vi "Explore_Volume.vi"(5 "Traverse line In":T1 {"Carrier_2 Q (l/min)" format="%#.2f"; "Row Duration (mins)" format="%#.1f"; "Row No" min=0; "Trace Gas Concentration (%)" min=0.0 format="%#_4f"; "Carrier_1 Q (l/min)" format="%#.4f"; "Start X" format="%#.2f"; "Start Y" format="%#.2f"; "Start Z" format="%#.2f"; "End X" format="%#.2f"; "End Y" format="%#.2f"; "End Z" format="%#.2f"; "Tunnel Speed" format="%#.2f"; "Averaging time (mins)" min=0.0 format="%#.2f"}) -> (0 "pointIDs":string[](array[string]), 2 "Position Array":sgl[][](array[numeric]))   [LabVIEW 2020]
uses:
  Traverse_cluster.ctl
  Spacing.ctl
  Controls/Multi_run_mode.ctl
panel:
  # "X           Y          Z"
  # "Start"
  # "End"
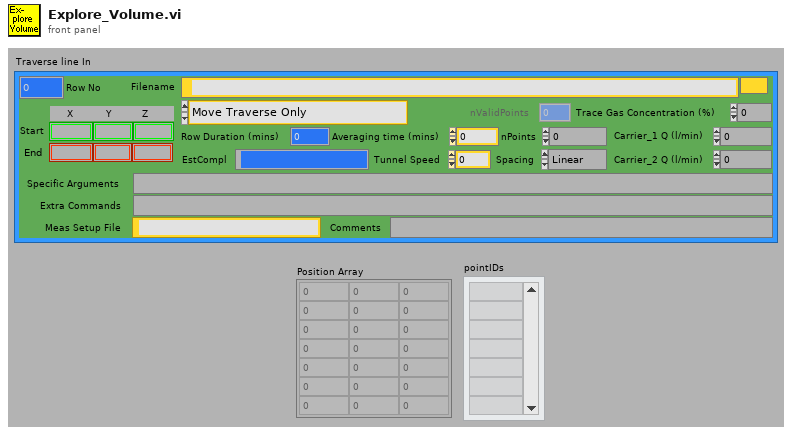
[diagram p1: front panel]
types:
  T1 = typedef "Traverse_cluster.ctl" = cluster{"Start X":sgl, "Start Y":sgl, "Start Z":sgl, "End X":sgl, "End Y":sgl, "End Z":sgl, "nPoints":i32, "Spacing":T2, "Filename":path, "Tunnel Speed":dbl, "Averaging time (mins)":dbl, "Extra Commands":string, "Carrier_1 Q (l/min)":dbl, "Carrier_2 Q (l/min)":dbl, "Trace Gas Concentration (%)":dbl, "Specific Arguments":string, "Comments":string, "Row No":i32, "Row Type Selector":T3, "EstCompl":string, "Row Duration (mins)":dbl, "nValidPoints":i32, "Meas Setup File":string}
  T2 = typedef "Spacing.ctl" = enum16{"Linear", "Log", "Gauss", "Specified", "N/A"}
  T3 = typedef "Multi_run_mode.ctl" = enum16{"Move Traverse Only", "Set Tunnel Speed Only", "Set Source Only", "Set Measurement Conditions", "Single Measurement", "Vertical Profile", "Lateral Profile", "Longitudinal Profile", "Multi-Axis Profile", "Explore Volume", "Auto Calibrate", "Meas Fast FID Bkgnd", "Check Beam Power", "Scanning Valve Measurement", "Run VI Named:", "Set ADAM Ch", "Wait (minutes)", "Send Message", "Synchronize With:", "Fall Back to this Row", "Turn Off Row Repeating", "Traverse 3D Volume", "Blank Row", "Jump to Fall Back Row"}
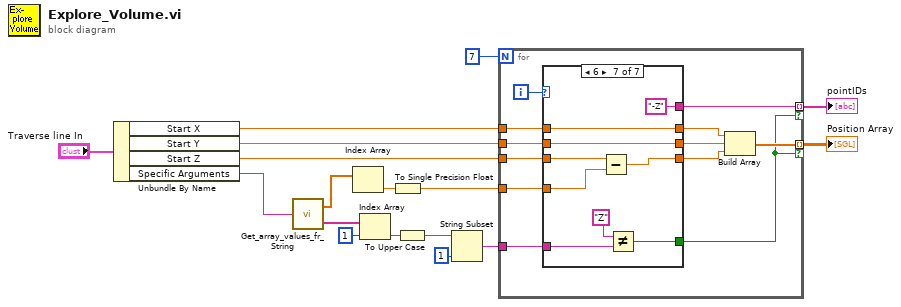
[diagram p0: block diagram]
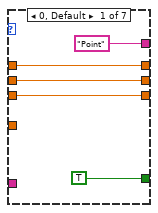
[diagram p2: hidden frame]
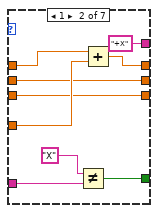
[diagram p3: hidden frame]
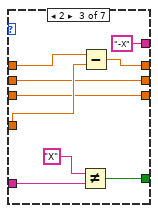
[diagram p4: hidden frame]
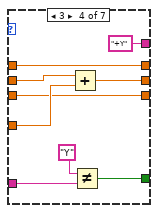
[diagram p5: hidden frame]
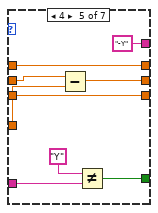
[diagram p6: hidden frame]
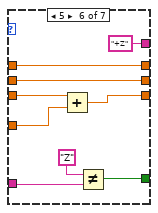
[diagram p7: hidden frame]
diagram:
  n1 = Unbundle By Name("Traverse line In") -> ("Start X"=w16:sgl, "Start Y"=w15:sgl, "Start Z"=w14:sgl, "Specific Arguments"=w12:string)
  n2 = call "Get_array_values_fr_String.vi"("String Value"=w12) -> ("Numeric Array"=w11:dbl[], "String array"=w9:string[])
  n3 = Index Array(array=w11) -> (element=w10:dbl)  [unwired: 1 in]
  n4 = Index Array(array=w9, index=1) -> (element=w7:string)
  n5 = To Single Precision Float(number=w10) -> (single precision float=w3:sgl)
  n6 = To Upper Case(1:w7) -> (0:w6:string)
  n7 = String Subset(string=w6, length (rest)=1 ("length (rest)")) -> (substring=w5:string)  [unwired: 1 in]
  n8 = for {
    N: 7 -> [_]
    tunnel: w16 -> [w28]
    tunnel: w15 -> [w27]
    tunnel: w14 -> [w26]
    tunnel: w3 -> [w25]
    tunnel: [w20] -> w2 mode=indexing if=w18
    tunnel: w5 -> [w24]
    tunnel: [w19] -> w1 mode=indexing if=w18
    i -> [w29]
    n9 = case shown="6" w29 {
      tunnel: w28 -> [w34 w42 w52 w59 w66 w75 w84]
      tunnel: [w34 w41 w51 w59 w66 w75 w84] -> w23
      tunnel: w27 -> [w33 w40 w49 w61 w70 w76 w85]
      tunnel: [w33 w40 w49 w57 w69 w76 w85] -> w22
      tunnel: w26 -> [w32 w39 w48 w58 w67 w79 w88]
      tunnel: [w32 w39 w48 w58 w67 w77 w86] -> w21
      tunnel: w25 -> [_ w43 w50 w60 w68 w78 w87]
      tunnel: [TRUE w36 w45 w54 w63 w72 w81] -> w18
      tunnel: w24 -> [_ w37 w47 w55 w64 w73 w82]
      tunnel: ["Point" "+X" "-X" "+Y" "-Y" "+Z" "-Z"] -> w19
      frame 0, Default {
      }
      frame 1 {
        n10 = Not Equal?(x="X", y=w37) -> (x != y?=w36:bool)
        n11 = Add(x=w42, y=w43) -> (x+y=w41:sgl)
      }
      frame 2 {
        n12 = Not Equal?(x="X", y=w47) -> (x != y?=w45:bool)
        n13 = Subtract(x=w52, y=w50) -> (x-y=w51:sgl)
      }
      frame 3 {
        n14 = Add(x=w61, y=w60) -> (x+y=w57:sgl)
        n15 = Not Equal?(x="Y", y=w55) -> (x != y?=w54:bool)
      }
      frame 4 {
        n16 = Subtract(x=w70, y=w68) -> (x-y=w69:sgl)
        n17 = Not Equal?(x="Y", y=w64) -> (x != y?=w63:bool)
      }
      frame 5 {
        n18 = Add(x=w79, y=w78) -> (x+y=w77:sgl)
        n19 = Not Equal?(x="Z", y=w73) -> (x != y?=w72:bool)
      }
      frame 6 {
        n20 = Subtract(x=w88, y=w87) -> (x-y=w86:sgl)
        n21 = Not Equal?(x="Z", y=w82) -> (x != y?=w81:bool)
      }
    }
    n22 = Build Array(w23, w22, w21) -> (w20:sgl[])
  }
  "Position Array" <- w2
  "pointIDs" <- w1
